vi "Msgbox - Release Q.vi"(8 "Error In":errorcluster) -> (0 "Error Out":errorcluster)   [LabVIEW 2013]
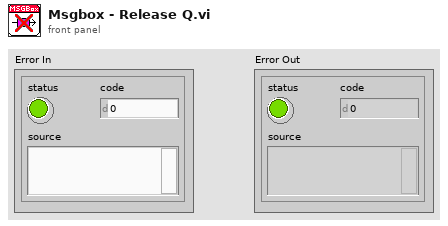
[diagram p1: front panel]
types:
  T1 = cluster{"Show":bool, "Priority":i32, "Message":string}
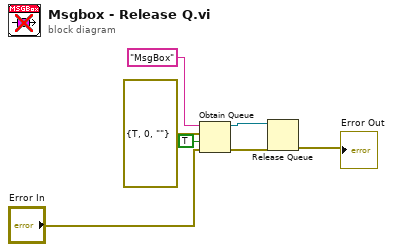
[diagram p0: block diagram]
diagram:
  n1 = Obtain Queue(name (unnamed)="MsgBox", element data type=T1 {"Show"=TRUE, "Priority"=0, "Message"=""}, create if not found? (T)=TRUE, error in (no error)="Error In") -> (queue out=w2:refnum<queue>, error out=w3:errorcluster)  [unwired: 1 in, 1 out]
  n2 = Release Queue(queue=w2, error in (no error)=w3) -> (error out=→"Error Out":errorcluster)  [unwired: 1 in, 2 out]
